vi "add element to sample.vi"(7 "sample size in":i32, 10 "element in":dbl, 11 "Array in":dbl[](array[numeric])) -> (3 "Array out":dbl[](array[numeric]))   [LabVIEW 2018, in "LV2Julia_core.lvlib"]
uses:
  LV2Julia_core.lvlib
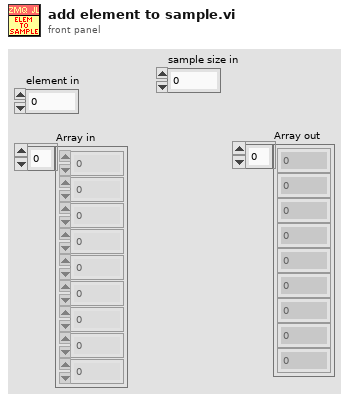
[diagram p1: front panel]
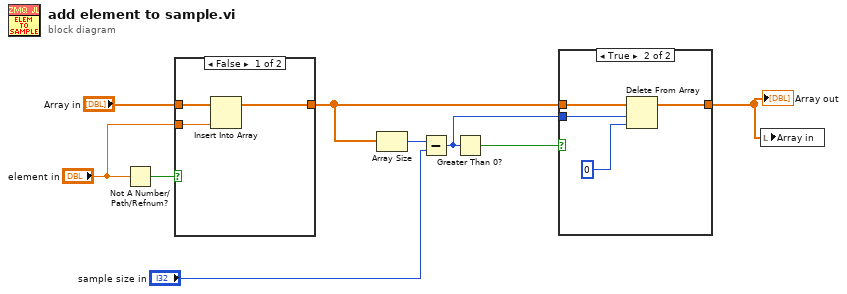
[diagram p0: block diagram]
diagram:
  n1 = Not A Number/Path/Refnum?(number/path/refnum="element in") -> (NaN/Path/Refnum?=w7:bool)
  n2 = case shown="False" w7 {
    tunnel: [w12 w13] -> w3
    tunnel: "Array in" -> [w11 w13]
    tunnel: "element in" -> [w10 _]
    frame False {
      n3 = Insert Into Array(array=w11, new element=w10) -> (w12:dbl[])  [unwired: 1 in]
    }
    frame True {
    }
  }
  n4 = Array Size(array=w3) -> (size(s)=w6:i32)
  n5 = Subtract(x=w6, y="sample size in") -> (x-y=w1:i32)
  n6 = Greater Than 0?(x=w1) -> (x > 0?=w4:bool)
  n7 = case shown="True" w4 {
    tunnel: w3 -> [w14 w18]
    tunnel: [w14 w15] -> w2
    tunnel: w1 -> [_ w16]
    frame False {
    }
    frame True {
      n8 = Delete From Array(array=w18, length=w16, index=0) -> (array with subset deleted=w15:dbl[])  [unwired: 1 out]
    }
  }
  "Array out" <- w2
  n9 = local write "Array in"(w2) -> ()
